vi "Read offset.vi"(8 "error in (no error)":errorcluster, 11 "Class 2 in":refnum<class "Class 2.lvclass">) -> (0 "error out":errorcluster, 2 "offset":u64, 3 "Class 2 out":refnum<class "Class 2.lvclass">)   [LabVIEW 2016, in "Data Sharing Framework.Runtime.lvlib" / "Class 2.lvclass"]
uses:
  Class 2.lvclass
  Class 2.lvclass/Class 2.ctl
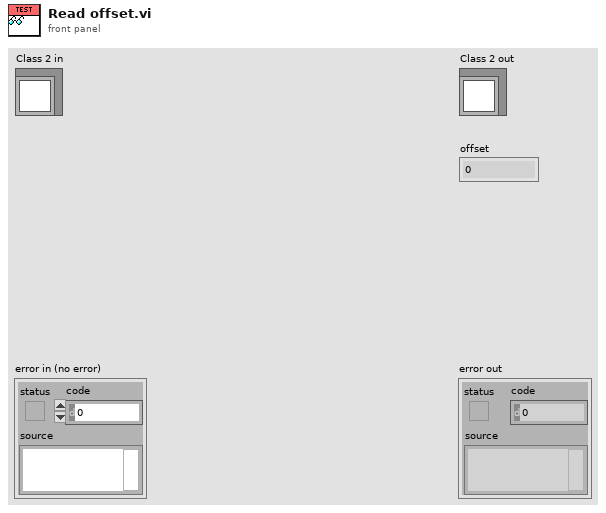
[diagram p1: front panel]
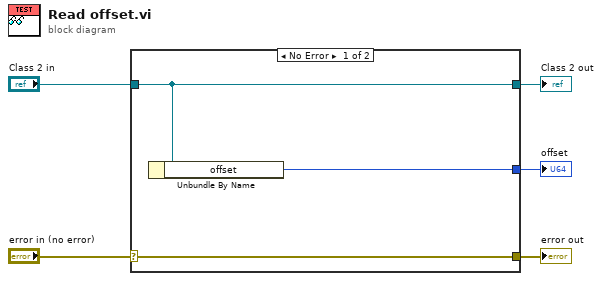
[diagram p0: block diagram]
diagram:
  n1 = case shown="No Error" "error in (no error)" {
    selector: "error in (no error)" -> [w8 w9]
    tunnel: [w8 w9] -> w4
    tunnel: [w7 w10] -> w2
    tunnel: "Class 2 in" -> [w7 w10]
    tunnel: [w6 _] -> w1
    frame No Error {
      n2 = Unbundle By Name(w7) -> ("offset"=w6:u64)
    }
    frame Error {
    }
  }
  "error out" <- w4
  "Class 2 out" <- w2
  "offset" <- w1
